vi "Configure Power.vi"(8 "error in (no error)":errorcluster, 10 "Power [dBm]":dbl, 11 "VNA-Keysight PNA in":refnum<class "VNA-Keysight PNA.lvclass">) -> (0 "error out":errorcluster, 3 "VNA-Keysight PNA out":refnum<class "VNA-Keysight PNA.lvclass">)   [LabVIEW 2020, in "VNA-Keysight PNA.lvclass"]
doc: "Configure the output power.\nThe power will be corrected to the nearest supported."
uses:
  VNA-Keysight PNA.lvclass
  C:/Sandbox/Git_Sandbox/WiSpry Test Framework source code (LV20)/WiSpry Test Framework/Instruments/Instrument.lvclass
  Instrument.lvclass/Instrument.ctl
  Instrument.lvclass
  <instrlib>/Keysight PNA Series/Keysight PNA Series.lvlib
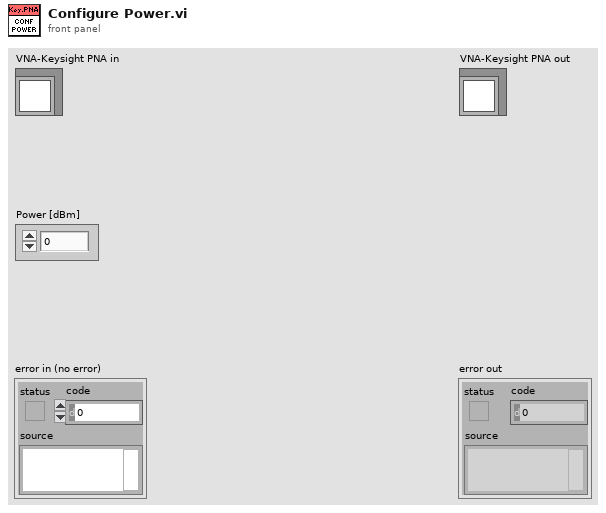
[diagram p1: front panel]
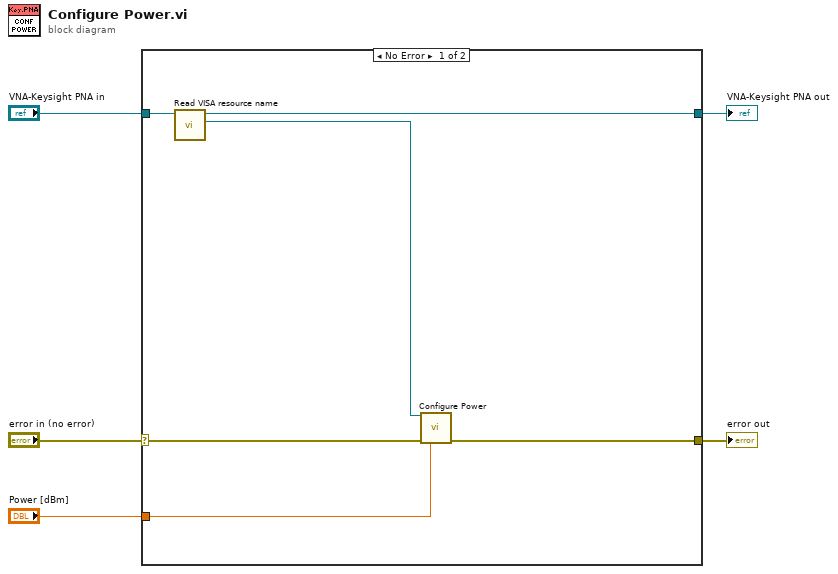
[diagram p0: block diagram]
diagram:
  n1 = case shown="No Error" "error in (no error)" {
    selector: "error in (no error)" -> [w9 w12]
    tunnel: [w10 w13] -> w3
    tunnel: "VNA-Keysight PNA in" -> [w11 w13]
    tunnel: [w8 w12] -> w4
    tunnel: "Power [dBm]" -> [w6 _]
    frame No Error {
      n2 = call "Read VISA resource name.vi"("Instrument in"=w11) -> ("VISA resource name"=w7:refnum<visa-resource-name>, "Instrument out"=w10:refnum<class "VNA-Keysight PNA.lvclass">)  [unwired: 9 in]
      n3 = call <instrlib>:"Configure Power.vi"("VISA resource name"=w7, "error in (no error)"=w9, "Power Level (0 dBm)"=w6) -> ("error out"=w8:errorcluster)  [unwired: 11 in, 1 out]
    }
    frame Error {
    }
  }
  "error out" <- w4
  "VNA-Keysight PNA out" <- w3
